vi "Create Waveform.vi"(0 "Max Waveform Size":i32, 5 "Sample Rate":dbl, 9 "Transient Configuration":T1={"Delay - t1 (s)"=10.0, "Duration of the pulse (s)"=10.0, "Delay - t2 (s)"=10.0, "Load Current 1 - Iload1 (A)"=1.0, "Load Current 2 - Iload2 (A)"=0.0, "Slew rate A/us"=0.001, "Fgen Voltage to Current Ratio"=1.0} {"Fgen Voltage to Current Ratio" min=1.0 format="%#_6p"}, 11 "error in":errorcluster) -> (4 "Waveform Graph":waveform(dbl)(graph), 15 "error out":errorcluster)   [LabVIEW 2020, in "LDO Load Transient_AWG.lvlib"]
uses:
  LDO Load Transient_AWG.lvlib
  Typedefs/Transient Configuration.ctl
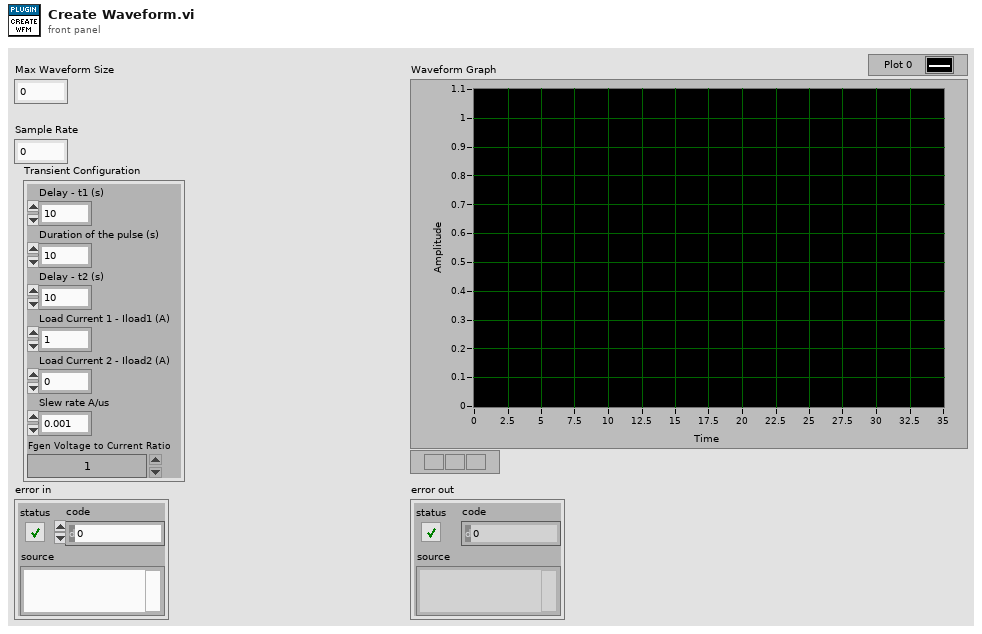
[diagram p1: front panel]
types:
  T1 = typedef "LDO Load Transient_AWG.lvlib/Transient Configuration.ctl" = cluster{"Delay - t1 (s)":dbl, "Duration of the pulse (s)":dbl, "Delay - t2 (s)":dbl, "Load Current 1 - Iload1 (A)":dbl, "Load Current 2 - Iload2 (A)":dbl, "Slew rate A/us":dbl, "Fgen Voltage to Current Ratio":dbl}
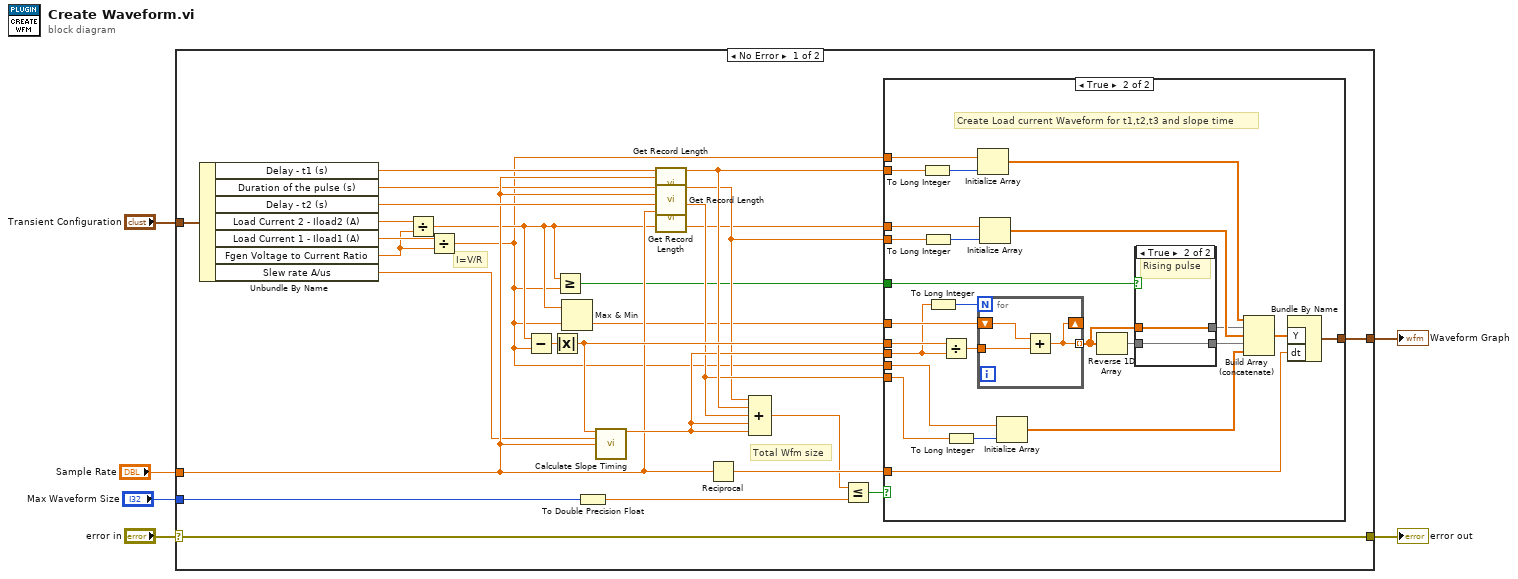
[diagram p0: block diagram]
diagram:
  n1 = case shown="No Error" "error in" {
    selector: "error in" -> [w22 w65]
    tunnel: [w27 _] -> w6
    tunnel: "Transient Configuration" -> [w25 _]
    tunnel: [w22 w65] -> w3
    tunnel: "Max Waveform Size" -> [w21 _]
    tunnel: "Sample Rate" -> [w17 _]
    frame No Error {
      # "I=V/R"
      # "Total Wfm size"
      n2 = Unbundle By Name(w25) -> ("Delay - t1 (s)"=w24:dbl, "Duration of the pulse (s)"=w16:dbl, "Delay - t2 (s)"=w20:dbl, "Load Current 2 - Iload2 (A)"=w10:dbl, "Load Current 1 - Iload1 (A)"=w12:dbl, "Fgen Voltage to Current Ratio"=w11:dbl, "Slew rate A/us"=w14:dbl)
      n3 = Divide(x=w10, y=w11) -> (x/y=w9:dbl)
      n4 = Divide(x=w12, y=w11) -> (x/y=w8:dbl)
      n5 = Subtract(x=w9, y=w8) -> (x-y=w32:dbl)
      n6 = Absolute Value(x=w32) -> (abs(x)=w29:dbl)
      n7 = Greater Or Equal?(x=w9, y=w8) -> (x >= y?=w7:bool)
      n8 = Max & Min(x=w9, y=w8) -> (min(x,y)=w13:dbl)  [unwired: 1 out]
      n9 = To Double Precision Float(number=w21) -> (double precision float=w15:dbl)
      n10 = call "Calculate Slope Timing.vi"("Current Difference"=w29, "Slew rate A/us"=w14, "Sample Rate"=w17) -> ("Slope Record Length"=w23:dbl)  [unwired: 12 in]
      n11 = call "Get Record Length.vi"("Time (s)"=w24, "Sample Rate"=w17) -> ("Record Length"=w28:dbl)  [unwired: 13 in]
      n12 = call "Get Record Length.vi"("Time (s)"=w16, "Sample Rate"=w17) -> ("Record Length"=w18:dbl)  [unwired: 13 in]
      n13 = call "Get Record Length.vi"("Time (s)"=w20, "Sample Rate"=w17) -> ("Record Length"=w19:dbl)  [unwired: 13 in]
      n14 = Reciprocal(x=w17) -> (1/x=w30:dbl)
      n15 = Compound Arithmetic op=ADD(w18, w28, w19, w23, w23) -> (w26:dbl)
      n16 = Less Or Equal?(x=w26, y=w15) -> (x <= y?=w31:bool)
      n17 = case shown="True" w31 {
        tunnel: w30 -> [_ w53]
        tunnel: w23 -> [_ w40]
        tunnel: w29 -> [_ w52]
        tunnel: w13 -> [_ w51]
        tunnel: w8 -> [_ w50]
        tunnel: w19 -> [_ w49]
        tunnel: w9 -> [_ w48]
        tunnel: w18 -> [_ w47]
        tunnel: w8 -> [_ w46]
        tunnel: w28 -> [_ w45]
        tunnel: [_ w44] -> w27
        tunnel: w7 -> [_ w37]
        frame False {
        }
        frame True {
          # "Create Load current Waveform for t1,t2,t3 and slope time"
          n18 = To Long Integer(number=w45) -> (32bit integer=w43:i32)
          n19 = To Long Integer(number=w47) -> (32bit integer=w42:i32)
          n20 = To Long Integer(number=w40) -> (32bit integer=w39:i32)
          n21 = Divide(x=w52, y=w40) -> (x/y=w55:dbl)
          n22 = To Long Integer(number=w49) -> (32bit integer=w41:i32)
          n23 = Initialize Array(w46, w43) -> (w54:dbl[])
          n24 = for {
            N: w39 -> [_]
            tunnel: w55 -> [w63]
            tunnel: [w62] -> w34 mode=indexing
            shift-right: [w62] -> _
            shift-left: w51 -> [w64]
            n25 = Add(x=w64, y=w63) -> (x+y=w62:dbl)
          }
          n26 = Initialize Array(w48, w42) -> (w57:dbl[])
          n27 = Initialize Array(w50, w41) -> (w56:dbl[])
          n28 = Reverse 1D Array(array=w34) -> (reversed array=w36:dbl[])
          n29 = case shown="True" w37 {
            tunnel: w36 -> [w59 w61]
            tunnel: [w58 w61] -> w35
            tunnel: w34 -> [w58 w60]
            tunnel: [w59 w60] -> w33
            frame False {
              # "Falling pulse"
            }
            frame True {
              # "Rising pulse"
            }
          }
          n30 = Build Array (concatenate)(w54, w33, w57, w35, w56) -> (w38:dbl[])
          n31 = Bundle By Name("Y"=w38, "dt"=w53) -> (w44:waveform(dbl))  [unwired: 1 in]
        }
      }
    }
    frame Error {
    }
  }
  "Waveform Graph" <- w6
  "error out" <- w3
